vi "Read List of Functions.vi"(8 "error in (no error)":errorcluster, 11 "List of Functions Message in":refnum<class "List of Functions Message.lvclass">) -> (0 "error out":errorcluster, 2 "List of Functions":string[](array[string]), 3 "List of Functions Message out":refnum<class "List of Functions Message.lvclass">)   [LabVIEW 2016, in "Controller UI.lvlib" / "List of Functions Message.lvclass"]
uses:
  <userlib>/Common Components/Controller UI/Messages/List of Functions Message/List of Functions Message.lvclass
  <userlib>/Common Components/Controller UI/Messages/List of Functions Message/List of Functions Message.lvclass/List of Functions Message.ctl
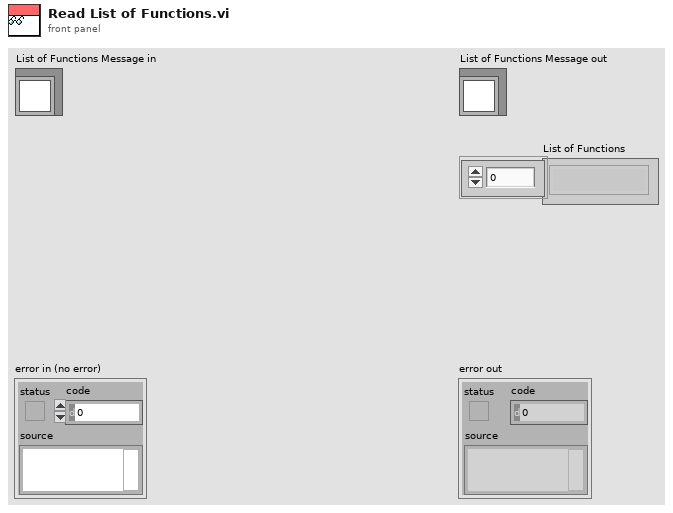
[diagram p1: front panel]
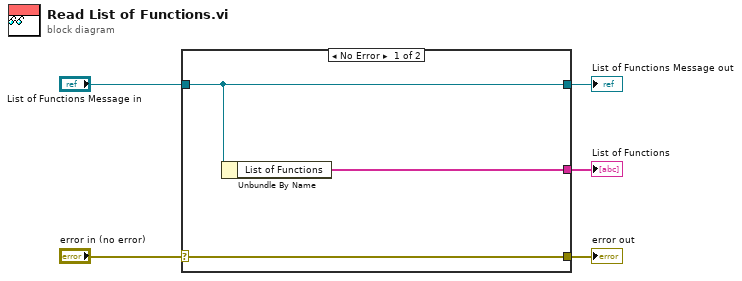
[diagram p0: block diagram]
diagram:
  n1 = case shown="No Error" "error in (no error)" {
    selector: "error in (no error)" -> [w8 w9]
    tunnel: [w8 w9] -> w4
    tunnel: [w7 w10] -> w2
    tunnel: "List of Functions Message in" -> [w7 w10]
    tunnel: [w6 _] -> w1
    frame No Error {
      n2 = Unbundle By Name(w7) -> ("List of Functions"=w6:string[])
    }
    frame Error {
    }
  }
  "error out" <- w4
  "List of Functions Message out" <- w2
  "List of Functions" <- w1
